vi "ReadXlsFile.vi"(0 "Robot ID":string, 1 "Motor ID":string) -> (2 "Can Bus ID":string, 3 "PWM Channel":string, 4 "PDP Channel ID":string)   [LabVIEW 2016]
uses:
  <vilib>/Utility/file.llb/Read Delimited Spreadsheet (string).vi
panel:
  out "Row with Info":i32
  out "Motor ID from Row x":string
  out "Number of Rows":i32
  out "Robot ID from Row x":string
  out "Number of Columns":i32
  out "subarray":string[](array[string])
  out "all rows":string[][](array[string])
  in  "file path (dialog if empty) 2":path=path "C:/git/ViTestFiles/RobotConfiguration-8.xml"
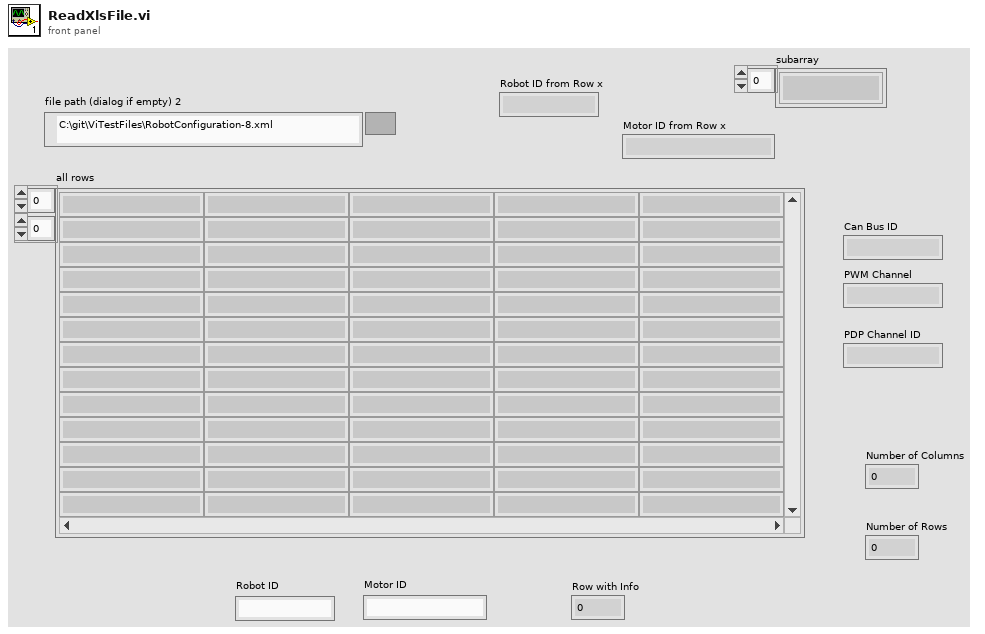
[diagram p1: front panel]
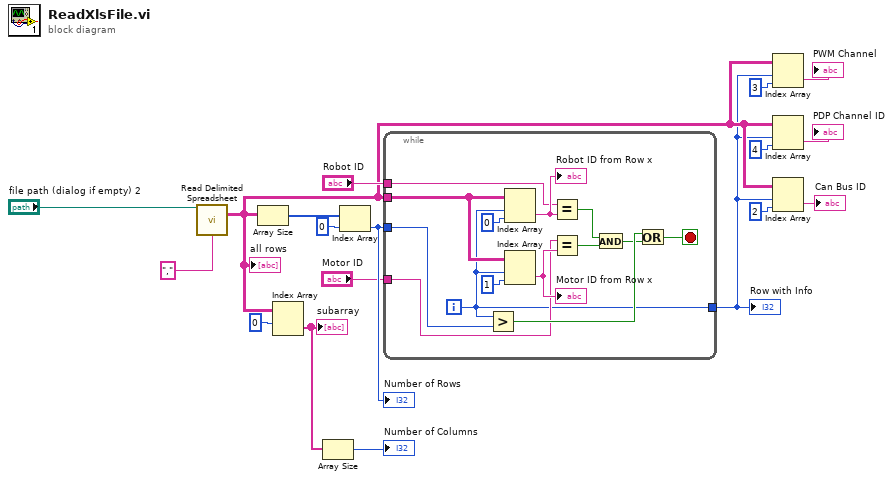
[diagram p0: block diagram]
diagram:
  n1 = call-poly <vilib>:"Read Delimited Spreadsheet.vi"("file path (dialog if empty)"="file path (dialog if empty) 2", "delimiter (\\t)"="," ("delimiter (\\t)")) -> ("all rows"=w8:string[][])  [unwired: 8 in, 5 out]
  "all rows" <- w8
  n2 = Array Size(array=w8) -> (size(s)=w13:i32[])
  n3 = Index Array(array=w8, index (row)=0) -> (element=w15:string[])  [unwired: 1 in]
  "subarray" <- w15
  n4 = Array Size(array=w15) -> (size(s)=→"Number of Columns":i32)
  n5 = Index Array(array=w13, index=0) -> (element=w11:i32)
  "Number of Rows" <- w11
  n6 = while {
    tunnel: w8 -> [w25]
    tunnel: w11 -> [w30]
    tunnel: "Robot ID" -> [w27]
    tunnel: "Motor ID" -> [w23]
    tunnel: [w19] -> w7
    i -> [w19]
    stop <- w29 stop-if-true
    n7 = Greater?(x=w19, y=w30) -> (0:w31:bool)
    n8 = Index Array(array=w25, index (row)=w19, index (col)=0 ("disabled index (col)")) -> (element=w28:string)
    "Robot ID from Row x" <- w28
    n9 = Index Array(array=w25, index (row)=w19, index (col)=1) -> (element=w24:string)
    "Motor ID from Row x" <- w24
    n10 = Equal?(x=w27, y=w28) -> (x = y?=w22:bool)
    n11 = Equal?(x=w23, y=w24) -> (x = y?=w21:bool)
    n12 = And(x=w22, y=w21) -> (x .and. y?=w20:bool)
    n13 = Or(x=w31, y=w20) -> (x .or. y?=w29:bool)
  }
  "Row with Info" <- w7
  n14 = Index Array(array=w8, index (row)=w7, index (col)=3 ("disabled index (col)")) -> (element=→"PWM Channel":string)
  n15 = Index Array(array=w8, index (row)=w7, index (col)=4 ("disabled index (col)")) -> (element=→"PDP Channel ID":string)
  n16 = Index Array(array=w8, index (row)=w7, index (col)=2 ("disabled index (col)")) -> (element=→"Can Bus ID":string)
